vi "Write ADU Packet.vi"(8 "error in":errorcluster, 9 "modbus data unit":refnum<class "Modbus Data Unit.lvclass">, 10 "protocol layer":refnum<class "Network Protocol.lvclass">, 11 "IP transmission data unit in":refnum<class "IP Data Unit.lvclass">) -> (0 "error out":errorcluster, 2 "protocol layer out":refnum<class "Network Protocol.lvclass">, 3 "IP transmission data unit out":refnum<class "IP Data Unit.lvclass">)   [LabVIEW 2021, in "IP Data Unit.lvclass"]
doc: "This uses the protocol layer to write a modbus packet to the bus, wrapped in the IP transmission data unit."
uses:
  IP Data Unit.lvclass
  D:/my_projects/projects/Algorithms/Labview/21/Modbus_v21/Transmission Data Unit/Transmission Data Unit.lvclass
  Network Protocol/Network Protocol.lvclass
  Modbus Data Unit/Modbus Data Unit.lvclass/Modbus Data Unit.ctl
  IP Data Unit.lvclass/IP Data Unit.ctl
  Transmission Data Unit.lvclass/Transmission Data Unit.ctl
  Modbus Data Unit/Modbus Data Unit.lvclass
  Transmission Data Unit.lvclass
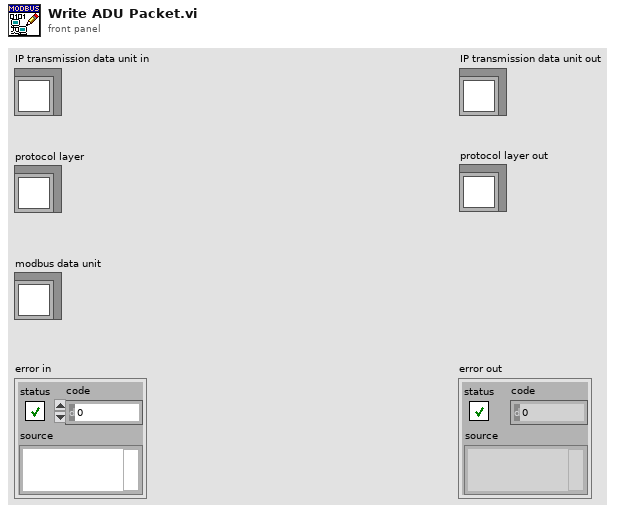
[diagram p1: front panel]
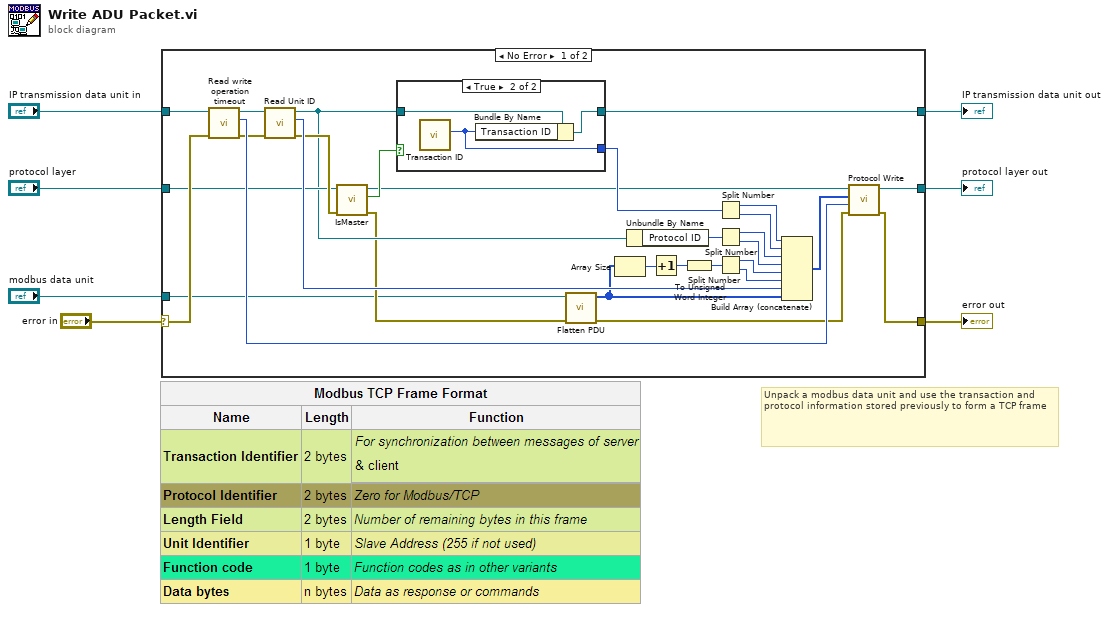
[diagram p0: block diagram]
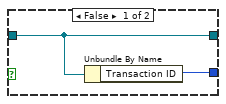
[diagram p2: hidden frame]
diagram:
  # "Unpack a modbus data unit and use the transaction and protocol information stored previously to form a TCP frame"
  n1 = case shown="No Error" "error in" {
    selector: "error in" -> [w20 w43]
    tunnel: [w37 w43] -> w1
    tunnel: "protocol layer" -> [w15 w44]
    tunnel: "modbus data unit" -> [w9 _]
    tunnel: [w36 w44] -> w4
    tunnel: "IP transmission data unit in" -> [w14 w45]
    tunnel: [w13 w45] -> w3
    frame No Error {
      n2 = call "Read write operation timeout.vi"("error in (no error)"=w20, "transmission data unit in"=w14) -> ("error out"=w22:errorcluster, "write operation timeout"=w23:i32, "transmission data unit out"=w21:refnum<class "IP Data Unit.lvclass">)  [unwired: 7 in]
      n3 = call "Read Unit ID.vi"("error in"=w22, "transmission data unit in"=w21) -> ("error out"=w19:errorcluster, "unit ID"=w24:u8, "transmission data unit out"=w12:refnum<class "IP Data Unit.lvclass">)  [unwired: 7 in]
      n4 = call-dynamic "IsMaster.vi"("error in (no error)"=w19, "Network Protocol in"=w15) -> ("error out"=w11:errorcluster, "isMaster"=w18:bool, "Network Protocol out"=w16:refnum<class "Network Protocol.lvclass">)  [unwired: 7 in]
      n5 = case shown="True" w18 {
        tunnel: w12 -> [w38 w42]
        tunnel: [w38 w41] -> w13
        tunnel: [w39 w40] -> w17
        frame False {
          n6 = Unbundle By Name(w38) -> ("Transaction ID"=w39:u16)
        }
        frame True {
          n7 = call "Transaction ID.vi"() -> ("Transaction ID"=w40:u16)  [unwired: 11 in]
          n8 = Bundle By Name(cluster=w42, "Transaction ID"=w40) -> (w41:refnum<class "IP Data Unit.lvclass">)
        }
      }
      n9 = call "Flatten PDU.vi"("error in"=w11, "modbus data unit in"=w9) -> ("error out"=w10:errorcluster, "Full modbus data unit"=w8:u8[])  [unwired: 8 in]
      n10 = Array Size(array=w8) -> (size(s)=w35:i32)
      n11 = Unbundle By Name(w12) -> ("Protocol ID"=w34:u16)
      n12 = Increment(x=w35) -> (x+1=w33:i32)
      n13 = To Unsigned Word Integer(number=w33) -> (unsigned 16bit integer=w32:u16)
      n14 = Split Number(x=w17) -> (hi(x)=w31:u8, lo(x)=w30:u8)
      n15 = Split Number(x=w34) -> (hi(x)=w29:u8, lo(x)=w28:u8)
      n16 = Split Number(x=w32) -> (hi(x)=w27:u8, lo(x)=w26:u8)
      n17 = Build Array (concatenate)(w31, w30, w29, w28, w27, w26, w24, w8) -> (w25:u8[])
      n18 = call-dynamic "Protocol Write.vi"("error in"=w10, "timeout"=w23, "data"=w25, "protocol layer in"=w16) -> ("error out"=w37:errorcluster, "protocol layer out"=w36:refnum<class "Network Protocol.lvclass">)  [unwired: 5 in, 1 out]
    }
    frame Error {
    }
  }
  "error out" <- w1
  "IP transmission data unit out" <- w3
  "protocol layer out" <- w4
